vi "Sensor_Globals.vi"() -> ()   [LabVIEW 2019]
panel:
  in  "Wheel_D_Angle (deg)":dbl
  in  "Wheel_C_Angle (deg)":dbl
  in  "Wheel_B_Angle (deg)":dbl
  in  "Wheel_A_Angle (deg)":dbl
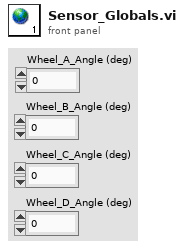
[diagram p1: front panel]
diagram:
